vi "BRig_arrTrig_CueAudio_L.vi"() -> (2 "output_CueAudio_L":i32)   [LabVIEW 2014]
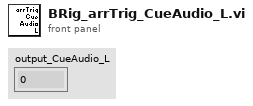
[diagram p1: front panel]
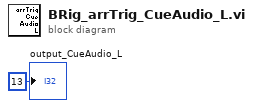
[diagram p0: block diagram]
diagram:
  "output_CueAudio_L" <- 13
